vi "Actor Core.vi"(8 "error in":errorcluster, 11 "Hot And Cold Source Unit View in":refnum<class "Hot And Cold Source Unit View.lvclass">) -> (0 "error out":errorcluster, 3 "Actor out":refnum<class "Actor.lvclass">)   [LabVIEW 2013, in "Hot And Cold Source Unit View.lvlib" / "Hot And Cold Source Unit View.lvclass"]
doc: "(<B>Filename</B>: Actor Framework.lvlib:Actor.lvclass:Actor Core.vi)\n\nReceives messages to the actor, reacts to them, and initiates any error handling that may shut the actor down.\n\nDescendant classes may override this VI to append parallel tasks for the actor to complete while it handles messages. Overrides use the Call Parent Method node."
uses:
  Hot And Cold Source Unit View.lvclass
  <vilib>/ActorFramework/Actor/Actor.lvclass
  Resources/UI Controls/Common/Side Button.ctl
  Hot And Cold Source Unit View.lvclass/Hot And Cold Source Unit View.ctl
  <vilib>/ActorFramework/Actor/Actor.lvclass/Actor.ctl
  <vilib>/ActorFrameworkMVC/View Actor/View Actor.lvclass
  <vilib>/ActorFramework/Message Enqueuer/Message Enqueuer.lvclass/Message Enqueuer.ctl
  Hot And Cold Source Unit View Messages/Set Test Node Map Msg/Set Test Node Map Msg.lvclass/Set Test Node Map Msg.ctl
  <vilib>/ActorFrameworkMVC/UI Controller Messages/Insert Subpanel Msg/Insert Subpanel Msg.lvclass/Insert Subpanel Msg.ctl
  <vilib>/ActorFrameworkMVC/UI Controller Messages/Move Subpanel Msg/Move Subpanel Msg.lvclass/Move Subpanel Msg.ctl
  Models/Hot And Cold Source Unit Model Messages/Set Parameters Map Msg/Set Parameters Map Msg.lvclass/Set Parameters Map Msg.ctl
  <vilib>/Utility/miscctls.llb/LVPositionTypeDef.ctl
  <vilib>/ActorFrameworkMVC/UI Controller Messages/Move Splitter Msg/Move Splitter Msg.lvclass/Move Splitter Msg.ctl
  Hot And Cold Source Unit View Messages/Get Channel List Msg/Get Channel List Msg.lvclass/Get Channel List Msg.ctl
  Hot And Cold Source Unit View Messages/Update Analysis Results Msg/Update Analysis Results Msg.lvclass/Update Analysis Results Msg.ctl
  <vilib>/ActorFramework/Message Enqueuer/Init from Existing Queue.vi
  <vilib>/ActorFramework/Message Enqueuer/Enqueue.vi
  <vilib>/ActorFramework/Message Priority Queue/Priority Enqueue.vi
  <vilib>/ActorFramework/Message Enqueuer/Message Enqueuer.lvclass
  Hot And Cold Source Unit View Messages/Initialize Parameters Msg/Initialize Parameters Msg.lvclass
  Hot And Cold Source Unit View Messages/Set Test Node Map Msg/Set Test Node Map Msg.lvclass
  Hot And Cold Source Unit View Messages/Update Test Node List Msg/Update Test Node List Msg.lvclass
  <vilib>/ActorFrameworkMVC/UI Controller Messages/Insert Subpanel Msg/Insert Subpanel Msg.lvclass
  <vilib>/ActorFrameworkMVC/UI Controller Messages/Move Subpanel Msg/Move Subpanel Msg.lvclass
  Models/Hot And Cold Source Unit Model Messages/Set Parameters Map Msg/Set Parameters Map Msg.lvclass
  Models/Hot And Cold Source Unit Model Messages/Analysis Msg/Analysis Msg.lvclass
  <vilib>/ActorFrameworkMVC/UI Controller Messages/Move Splitter Msg/Move Splitter Msg.lvclass
  Models/HVAC System Model Messages/Initialize Page Number Msg/Initialize Page Number Msg.lvclass
  Models/HVAC System Model Messages/Preview HVAC Msg/Preview HVAC Msg.lvclass
  Models/HVAC System Model Messages/Update Tiles Info Msg/Update Tiles Info Msg.lvclass
  Models/HVAC System Model Messages/Update Previous Button Visibility Msg/Update Previous Button Visibility Msg.lvclass
  Models/HVAC System Model Messages/Update Next Button Visibility Msg/Update Next Button Visibility Msg.lvclass
  Hot And Cold Source Unit View Messages/Get Channel List Msg/Get Channel List Msg.lvclass
  Hot And Cold Source Unit View Messages/Update Analysis Results Msg/Update Analysis Results Msg.lvclass
  Common/Control Reference/Control Reference.lvlib
  Common/File IO/File IO.lvlib
  <vilib>/ActorFrameworkMVC/UI Controller Messages/Get Model Actor Enqueuer Msg/Get Model Actor Enqueuer Msg.lvclass
  Resources/UI Controls/UI Control.lvlib
panel:
  in  "Cancel":bool
  out "Tab Control":enum32{"Parameters", "Result Analysis"}(tab)
  in  "N Channel":u16(ring)
  in  "N Node":u16(ring) caption="机组瞬时功率："
  in  "N Value":string
  in  "TCout Channel":u16(ring)
  in  "TCout Node":u16(ring) caption="冷凝器出水温度："
  in  "TCout Value":string
  in  "TCin Channel":u16(ring)
  in  "TCin Node":u16(ring) caption="冷凝器进水温度："
  in  "TCin Value":string
  in  "TEout Channel":u16(ring)
  in  "TEout Node":u16(ring) caption="蒸发器出水温度："
  in  "TEout Value":string
  in  "TEin Channel":u16(ring)
  in  "TEin Node":u16(ring) caption="蒸发器进水温度："
  in  "TEin Value":string
  in  "FC Channel":u16(ring)
  in  "FC Node":u16(ring) caption="冷凝器流量："
  in  "FC Value":string
  in  "FE Channel":u16(ring)
  in  "FE Node":u16(ring) caption="蒸发器流量："
  in  "FE Value":string
  out "Q0E Result":string caption="供冷量："
  out "Q0C Result":string caption="供冷量："
  out "FE Result":string caption="蒸发器流量："
  out "FC Result":string caption="冷凝器流量："
  out "TEin Result":string caption="蒸发器进水温度："
  out "TEout Result":string caption="蒸发器出水温度："
  out "TCin Result":string caption="冷凝器进水温度："
  out "TCout Result":string caption="冷凝器出水温度："
  in  "Analysis":bool
  in  "Side Buttons":enum32{"Parameters", "Result Analysis"}(radio)
  # "冷热源机组实际效能比"
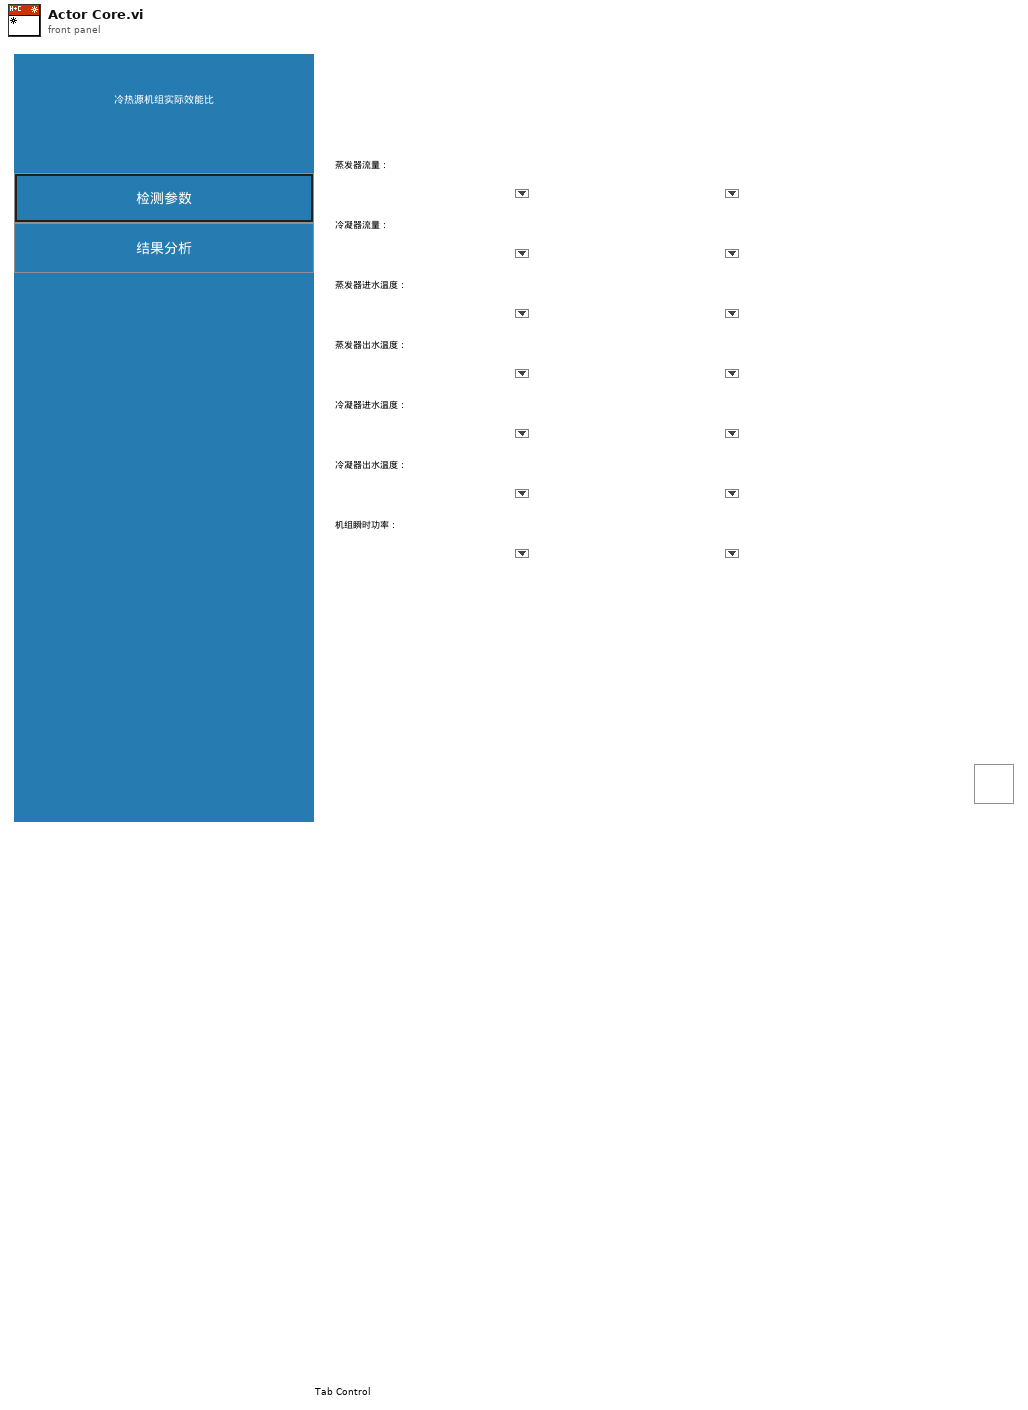
[diagram p1: front panel]
types:
  T1 = typedef "Hot And Cold Source Unit View.lvlib/Hot And Cold Source Unit View.lvclass/Events.ctl" = cluster{"Reinitialize All":refnum<user-event>, "Update Test Node Map":refnum<user-event>, "Update Results":refnum<user-event>}
  T2 = typedef "LVPositionTypeDef.ctl" = cluster{"Left":i32, "Top":i32}
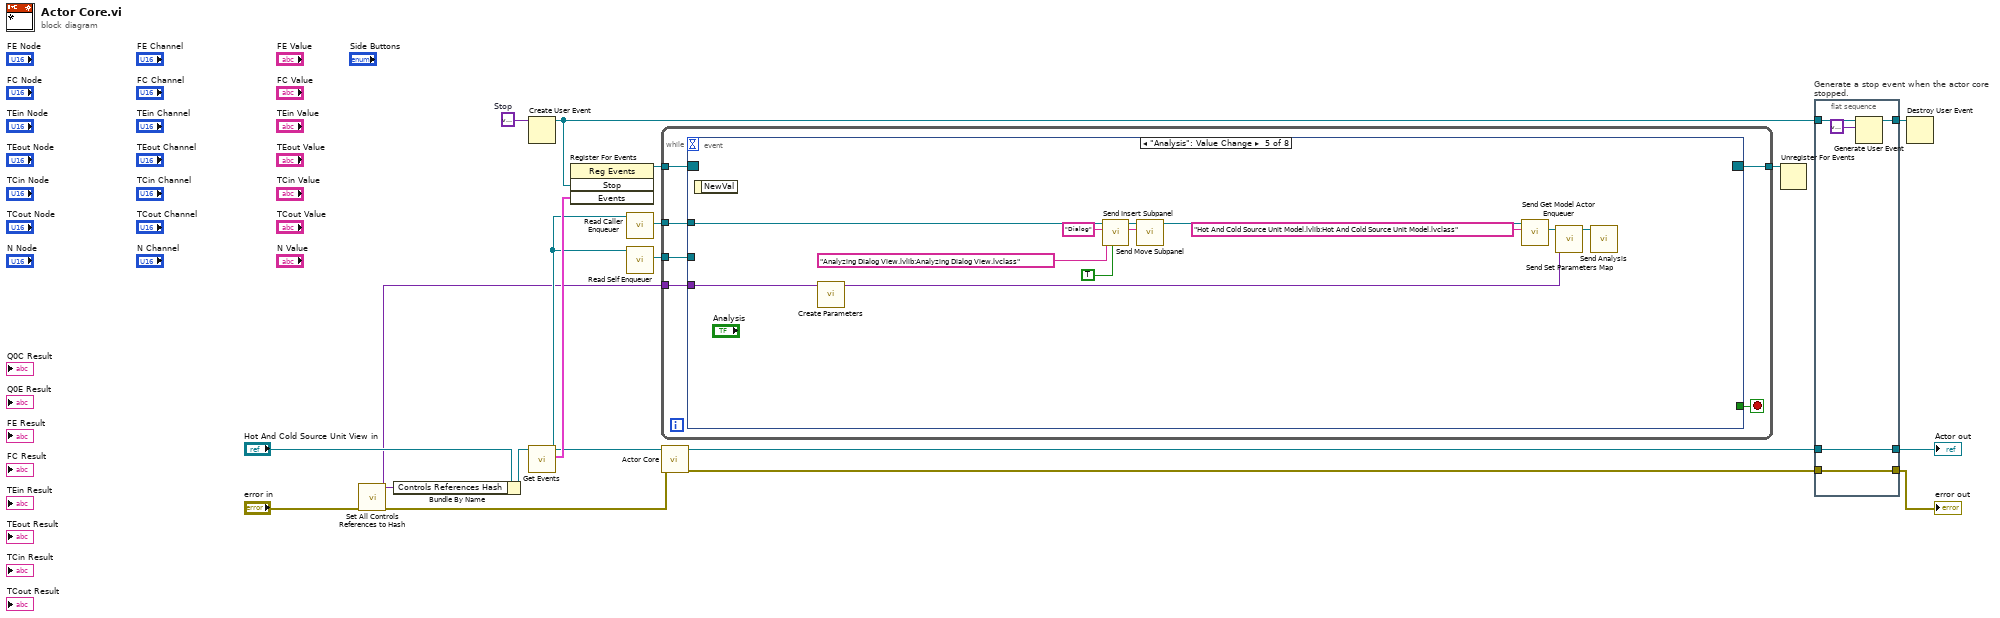
[diagram p0: block diagram]
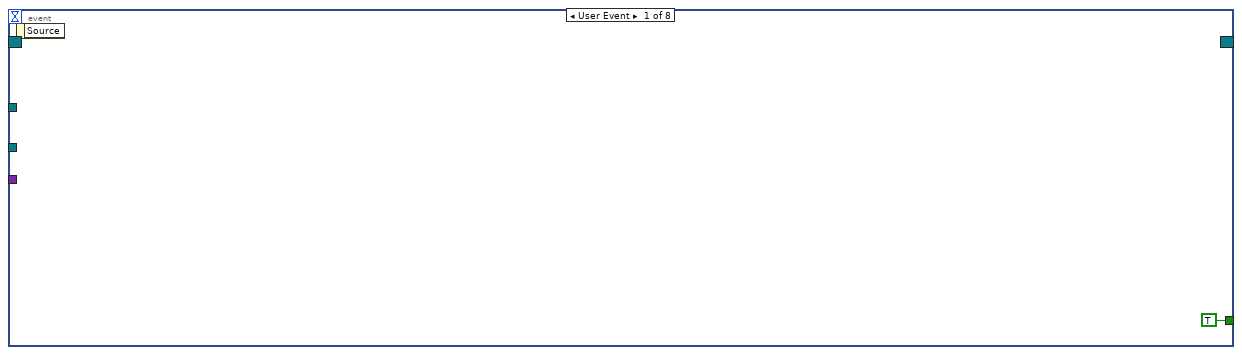
[diagram p2: hidden frame]
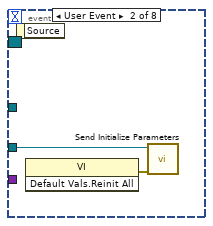
[diagram p3: hidden frame]
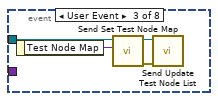
[diagram p4: hidden frame]
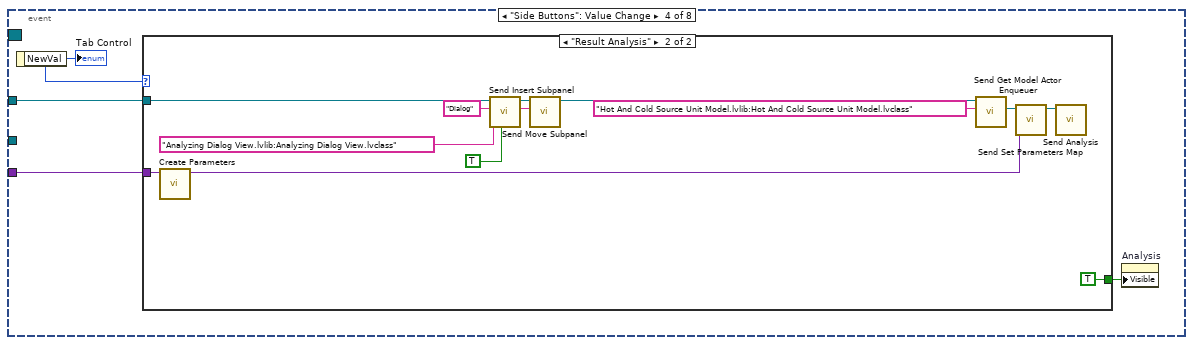
[diagram p5: hidden frame]
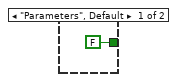
[diagram p6: hidden frame]
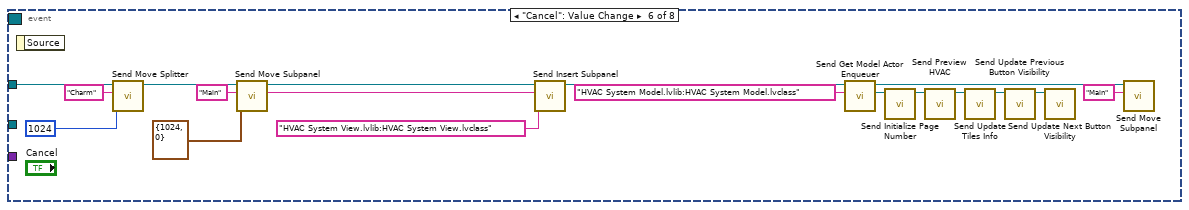
[diagram p7: hidden frame]
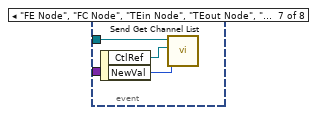
[diagram p8: hidden frame]
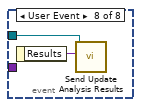
[diagram p9: hidden frame]
diagram:
  w18 = variant  # Stop
  n1 = call "Set All Controls References to Hash.vi"("error in (no error)"="error in") -> ("error out"=w3:errorcluster, "controls references hash"=w1:variant)  [unwired: 9 in]
  n2 = Bundle By Name(cluster="Hot And Cold Source Unit View in", "Controls References Hash"=w1) -> (w4:refnum<class "Hot And Cold Source Unit View.lvclass">)
  n3 = Create User Event(user event datatype=w18) -> (user event=w11:refnum<user-event>)  [unwired: 1 in, 1 out]
  n4 = call "Get Events.vi"("Hot And Cold Source Unit View in"=w4) -> ("Events"=w10:T1, "Hot And Cold Source Unit View out"=w8:refnum<class "Hot And Cold Source Unit View.lvclass">)  [unwired: 9 in]
  n5 = register-events(w11, w10) -> (reference out=w12:refnum<event-registration>)  [unwired: 2 in, 1 out]
  n6 = call <vilib>:"Read Caller Enqueuer.vi"("Actor"=w8) -> ("Caller Enqueuer"=w7:refnum<class "Message Enqueuer.lvclass">)  [unwired: 10 in]
  n7 = call <vilib>:"Read Self Enqueuer.vi"("Actor"=w8) -> ("Self Enqueuer"=w6:refnum<class "Message Enqueuer.lvclass">)  [unwired: 10 in]
  n8 = while {
    tunnel: [w24] -> w9
    tunnel: w12 -> [w22]
    tunnel: w7 -> [w21]
    tunnel: w6 -> [w20]
    tunnel: w1 -> [w19]
    stop <- w23 stop-if-true
    n9 = event shown="[4] \"Analysis\": Value Change" {
      selector: w22 -> [_ _ _ _ _ _ _ _]
      dyn-events: [_ _ _ _ _ _ _ _] -> w24
      timeout: _ -> [_ _ _ _ _ _ _ _]
      tunnel: [TRUE _ _ _ _ _ _ _] -> w23
      tunnel: w21 -> [_ _ _ w34 w59 w60 _ _]
      tunnel: w20 -> [_ w27 w31 _ _ _ w79 w80]
      tunnel: w19 -> [_ _ _ w33 w58 _ _ _]
      event User Event {
        n10 = event-data() -> ()  [unwired: 1 in, 1 out]
      }
      event User Event {
        n11 = event-data() -> ()  [unwired: 1 in, 1 out]
        n12 = invoke class="VI" method="Default Vals.Reinit All"() -> (error out=w26:errorcluster)  [unwired: 3 in, 2 out]
        n13 = call "Send Initialize Parameters.vi"("error in (no error)"=w26, "Message Enqueuer"=w27) -> ()  [unwired: 8 in, 2 out]
      }
      event User Event {
        n14 = event-data() -> ("Test Node Map"=w30:variant)  [unwired: 1 in]
        n15 = call "Send Set Test Node Map.vi"("Test Node Map"=w30, "Message Enqueuer"=w31) -> ("error out"=w28:errorcluster, "Message Enqueuer out"=w29:refnum<class "Message Enqueuer.lvclass">)  [unwired: 8 in]
        n16 = call "Send Update Test Node List.vi"("error in (no error)"=w28, "Message Enqueuer"=w29) -> ()  [unwired: 8 in, 2 out]
      }
      event "Side Buttons": Value Change {
        n17 = event-data() -> ("NewVal"=w35:enum32{"Parameters", "Result Analysis"})  [unwired: 1 in]
        "Tab Control" <- w35
        n18 = case shown="\"Result Analysis\"" w35 {
          tunnel: w34 -> [_ w48]
          tunnel: w33 -> [_ w44]
          tunnel: [FALSE TRUE] -> w32
          frame "Parameters", Default {
          }
          frame "Result Analysis" {
            w39 = "Dialog" ("Subpanel Name")
            n19 = call "Create Parameters.vi"("Controls References Hash"=w44) -> ("Parameters Map"=w43:variant)  [unwired: 9 in, 1 out]
            n20 = call <vilib>:"Send Insert Subpanel.vi"("Transparent? (F)"=TRUE, "View Name"="Analyzing Dialog View.lvlib:Analyzing Dialog View.lvclass", "Subpanel Name"=w39, "Message Enqueuer"=w48) -> ("Message Enqueuer out"=w42:refnum<class "Message Enqueuer.lvclass">)  [unwired: 6 in, 1 out]
            n21 = call <vilib>:"Send Move Subpanel.vi"("Subpanel Name"=w39, "Message Enqueuer"=w42) -> ("Message Enqueuer out"=w40:refnum<class "Message Enqueuer.lvclass">)  [unwired: 8 in, 1 out]
            n22 = call <vilib>:"Send Get Model Actor Enqueuer.vi"("Model Name"="Hot And Cold Source Unit Model.lvlib:Hot And Cold Source Unit Model.lvclass", "Message Enqueuer in"=w40) -> ("Reply"=w47:refnum<class "Message Enqueuer.lvclass">)  [unwired: 6 in, 3 out]
            n23 = call "Send Set Parameters Map.vi"("Parameters Map"=w43, "Message Enqueuer"=w47) -> ("Message Enqueuer out"=w46:refnum<class "Message Enqueuer.lvclass">)  [unwired: 8 in, 1 out]
            n24 = call "Send Analysis.vi"("Message Enqueuer"=w46) -> ()  [unwired: 9 in, 2 out]
          }
        }
        n25 = property on="Analysis" class="Bool"("Visible"=w32) -> ()  [unwired: 2 in, 2 out]
      }
      event "Analysis": Value Change {
        w50 = "Dialog" ("Subpanel Name")
        n26 = event-data() -> ()  [unwired: 1 in, 1 out]
        n27 = call "Create Parameters.vi"("Controls References Hash"=w58) -> ("Parameters Map"=w54:variant)  [unwired: 9 in, 1 out]
        n28 = call <vilib>:"Send Insert Subpanel.vi"("Transparent? (F)"=TRUE, "View Name"="Analyzing Dialog View.lvlib:Analyzing Dialog View.lvclass", "Subpanel Name"=w50, "Message Enqueuer"=w59) -> ("Message Enqueuer out"=w53:refnum<class "Message Enqueuer.lvclass">)  [unwired: 6 in, 1 out]
        n29 = call <vilib>:"Send Move Subpanel.vi"("Subpanel Name"=w50, "Message Enqueuer"=w53) -> ("Message Enqueuer out"=w51:refnum<class "Message Enqueuer.lvclass">)  [unwired: 8 in, 1 out]
        n30 = call <vilib>:"Send Get Model Actor Enqueuer.vi"("Model Name"="Hot And Cold Source Unit Model.lvlib:Hot And Cold Source Unit Model.lvclass", "Message Enqueuer in"=w51) -> ("Reply"=w57:refnum<class "Message Enqueuer.lvclass">)  [unwired: 6 in, 3 out]
        n31 = call "Send Set Parameters Map.vi"("Parameters Map"=w54, "Message Enqueuer"=w57) -> ("Message Enqueuer out"=w56:refnum<class "Message Enqueuer.lvclass">)  [unwired: 8 in, 1 out]
        n32 = call "Send Analysis.vi"("Message Enqueuer"=w56) -> ()  [unwired: 9 in, 2 out]
      }
      event "Cancel": Value Change {
        w71 = "Main" ("Subpanel Name")
        n33 = event-data() -> ()  [unwired: 1 in, 1 out]
        n34 = call <vilib>:"Send Move Splitter.vi"("Splitter Position"=1024, "Splitter Name"="Charm", "Message Enqueuer"=w60) -> ("Message Enqueuer out"=w61:refnum<class "Message Enqueuer.lvclass">)  [unwired: 7 in, 1 out]
        n35 = call <vilib>:"Send Move Subpanel.vi"("Position (0,0)"=T2 {"Left"=1024, "Top"=0}, "Subpanel Name"=w71, "Message Enqueuer"=w61) -> ("Message Enqueuer out"=w74:refnum<class "Message Enqueuer.lvclass">)  [unwired: 7 in, 1 out]
        n36 = call <vilib>:"Send Insert Subpanel.vi"("View Name"="HVAC System View.lvlib:HVAC System View.lvclass" ("Subpanel Name"), "Subpanel Name"=w71, "Message Enqueuer"=w74) -> ("Message Enqueuer out"=w69:refnum<class "Message Enqueuer.lvclass">)  [unwired: 7 in, 1 out]
        n37 = call <vilib>:"Send Get Model Actor Enqueuer.vi"("Model Name"="HVAC System Model.lvlib:HVAC System Model.lvclass", "Message Enqueuer in"=w69) -> ("Reply"=w66:refnum<class "Message Enqueuer.lvclass">, "Message Enqueuer out"=w68:refnum<class "Message Enqueuer.lvclass">)  [unwired: 6 in, 2 out]
        n38 = call "Send Initialize Page Number.vi"("Message Enqueuer"=w66) -> ("Message Enqueuer out"=w65:refnum<class "Message Enqueuer.lvclass">)  [unwired: 9 in, 1 out]
        n39 = call "Send Preview HVAC.vi"("Message Enqueuer"=w65) -> ("Message Enqueuer out"=w64:refnum<class "Message Enqueuer.lvclass">)  [unwired: 9 in, 1 out]
        n40 = call "Send Update Tiles Info.vi"("Message Enqueuer"=w64) -> ("Message Enqueuer out"=w63:refnum<class "Message Enqueuer.lvclass">)  [unwired: 9 in, 1 out]
        n41 = call "Send Update Previous Button Visibility.vi"("Message Enqueuer"=w63) -> ("Message Enqueuer out"=w62:refnum<class "Message Enqueuer.lvclass">)  [unwired: 9 in, 1 out]
        n42 = call "Send Update Next Button Visibility.vi"("Message Enqueuer"=w62) -> ()  [unwired: 9 in, 2 out]
        n43 = call <vilib>:"Send Move Subpanel.vi"("Subpanel Name"="Main", "Message Enqueuer"=w68) -> ()  [unwired: 8 in, 2 out]
      }
      event "FE Node", "FC Node", "TEin Node", "TEout Node", "TCin Node", "TCout Node", "N Node": Value Change {
        n44 = event-data() -> ("CtlRef"=w78:refnum<vi>, "NewVal"=w77:u16)  [unwired: 1 in]
        n45 = call "Send Get Channel List.vi"("Control Value"=w77, "Control Reference"=w78, "Message Enqueuer"=w79) -> ()  [unwired: 7 in, 2 out]
      }
      event User Event {
        n46 = event-data() -> ("Results"=w81:variant)  [unwired: 1 in]
        n47 = call "Send Update Analysis Results.vi"("Results"=w81, "Message Enqueuer"=w80) -> ()  [unwired: 8 in, 2 out]
      }
    }
  }
  n48 = call-parent "Actor Core.vi"("error in"=w3, "View Actor in"=w8) -> ("error out"=w15:errorcluster, "Actor out"=w16:refnum<class "Actor.lvclass">)  [unwired: 8 in]
  n49 = Unregister For Events(event registration refnum=w9) -> ()  [unwired: 1 in, 1 out]
  n50 = flat-sequence "Generate a stop event when the actor core stopped." {
    tunnel: w11 -> [w86]
    tunnel: [w84] -> w17
    tunnel: w16 -> [w83]
    tunnel: w15 -> [w82]
    tunnel: [w83] -> w14
    tunnel: [w82] -> w13
    frame #0 {
      n51 = Generate User Event(user event=w86, event data cluster=variant ("event data")) -> (user event out=w84:refnum<user-event>)  [unwired: 2 in, 1 out]
    }
  }
  n52 = Destroy User Event(user event=w17) -> ()  [unwired: 1 in, 1 out]
  "error out" <- w13
  "Actor out" <- w14
